vi "匹配FF01.vi"(1 "连接ID":refnum<k5>) -> (0 "匹配FF01":string)   [LabVIEW 2015]
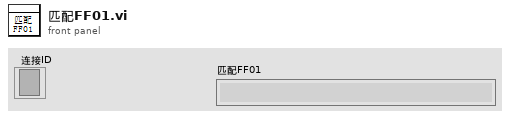
[diagram p1: front panel]
types:
  T1 = enum16{"匹配FF", "匹配01", "3", "4", "5", "6", "7", "8", "9"}
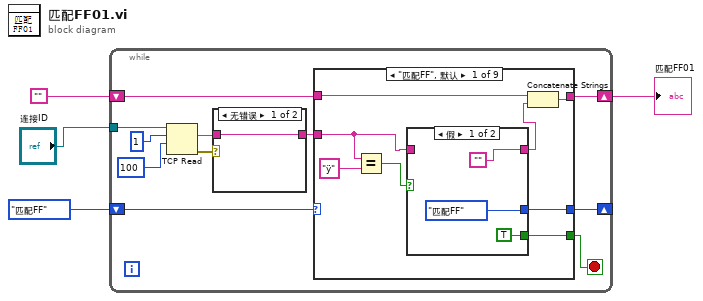
[diagram p0: block diagram]
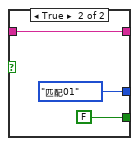
[diagram p2: hidden frame]
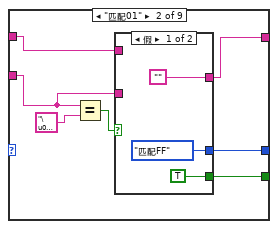
[diagram p3: hidden frame]
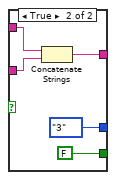
[diagram p4: hidden frame]
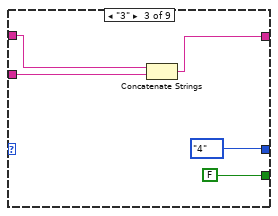
[diagram p5: hidden frame]
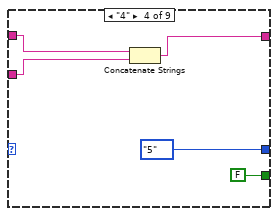
[diagram p6: hidden frame]
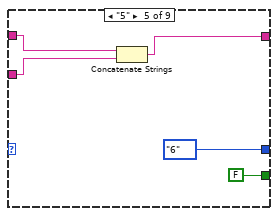
[diagram p7: hidden frame]
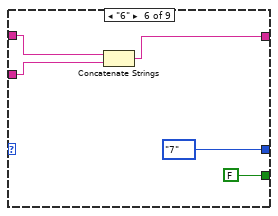
[diagram p8: hidden frame]
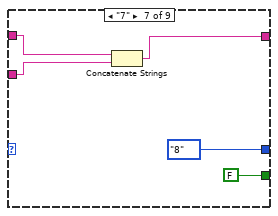
[diagram p9: hidden frame]
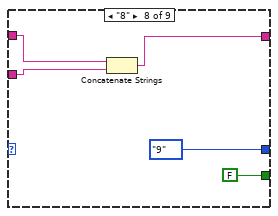
[diagram p10: hidden frame]
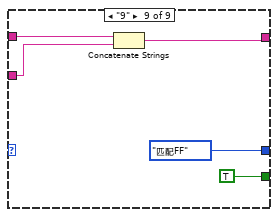
[diagram p11: hidden frame]
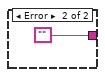
[diagram p12: hidden frame]
diagram:
  n1 = while {
    tunnel: "连接ID" -> [w15]
    shift-right: [w13] -> _
    shift-left: T1."匹配FF" -> [w14]
    shift-right: [w11] -> w2
    shift-left: "" -> [w12]
    stop <- w5 stop-if-true
    n2 = TCP Read(connection ID=w15, bytes to read=1, 9:100) -> (data out=w8:string, error out=w7:errorcluster)  [unwired: 2 in, 1 out]
    n3 = case shown="无错误" w7 {
      tunnel: w8 -> [w80 _]
      tunnel: [w80 ""] -> w6
      frame No Error {
      }
      frame Error {
      }
    }
    n4 = case shown="\"匹配FF\", 默认" w14 {
      tunnel: w6 -> [w21 w33 w48 w53 w58 w63 w68 w73 w78]
      tunnel: [w17 w31 w47 w52 w57 w62 w67 w72 w77] -> w11
      tunnel: [w20 w34 T1."4" T1."5" T1."6" T1."7" T1."8" T1."9" T1."匹配FF"] -> w13
      tunnel: w12 -> [w19 w32 w49 w54 w59 w64 w69 w74 w79]
      tunnel: [w16 w30 FALSE FALSE FALSE FALSE FALSE FALSE TRUE] -> w5
      frame "匹配FF", Default {
        n5 = Equal?(x=w21, y="ÿ") -> (x = y?=w22:bool)
        n6 = case shown="假" w22 {
          tunnel: w21 -> [_ w29]
          tunnel: ["" w29] -> w18
          tunnel: [T1."匹配FF" T1."匹配01"] -> w20
          tunnel: [TRUE FALSE] -> w16
          frame False {
          }
          frame True {
          }
        }
        n7 = Concatenate Strings(w19, w18) -> (w17:string)
      }
      frame "匹配01" {
        n8 = Equal?(x=w33, y="\u0001") -> (x = y?=w35:bool)
        n9 = case shown="假" w35 {
          tunnel: [T1."匹配FF" T1."3"] -> w34
          tunnel: w33 -> [_ w42]
          tunnel: ["" w41] -> w31
          tunnel: w32 -> [_ w43]
          tunnel: [TRUE FALSE] -> w30
          frame False {
          }
          frame True {
            n10 = Concatenate Strings(w43, w42) -> (w41:string)
          }
        }
      }
      frame "3" {
        n11 = Concatenate Strings(w49, w48) -> (w47:string)
      }
      frame "4" {
        n12 = Concatenate Strings(w54, w53) -> (w52:string)
      }
      frame "5" {
        n13 = Concatenate Strings(w59, w58) -> (w57:string)
      }
      frame "6" {
        n14 = Concatenate Strings(w64, w63) -> (w62:string)
      }
      frame "7" {
        n15 = Concatenate Strings(w69, w68) -> (w67:string)
      }
      frame "8" {
        n16 = Concatenate Strings(w74, w73) -> (w72:string)
      }
      frame "9" {
        n17 = Concatenate Strings(w79, w78) -> (w77:string)
      }
    }
  }
  "匹配FF01" <- w2
